vi "RGseriesSerialTest_voltage2.vi"() -> ()   [LabVIEW 2015]
uses:
  <vilib>/Platform/TimedLoop/XDataNode/timing_clust.ctl
  <vilib>/Platform/TimedLoop/XDataNode/nitl_modes.ctl
  <vilib>/Platform/TimedLoop/XDataNode/wakeup.ctl
  <vilib>/Instr/_visa.llb/VISA Configure Serial Port (Instr).vi
  <vilib>/platform/TimedLoop/XDataNode/XDataNode.xnode
  <vilib>/Platform/TimedLoop/XDataNode/XDNodeRunTimeDep.lvlib
panel:
  out "read buffer":string
  in  "Imax":dbl=1.0
  in  "stop":bool
  out "return count 8":u32
  out "return count 7":u32
  out "return count 6":u32
  out "return count 5":u32
  out "ICN MES A":dbl
  out "VCN MES V":dbl
  out "return count 4":u32
  out "return count 3":u32
  out "return count 2":u32
  out "return count":u32
  out "VCN MES":string
  in  "VISA resource name":refnum<visa-resource-name>="COM12"
  in  "timeout (10sec)":u32=10000
  out "ICN MES":string
  out "VCN_REQ_COM":string
  out "ICN_REQ_COM":string
  in  "VCN_REQ":dbl(knob) scale=0.0..5.0
  # "COM25"
  # "COM12"
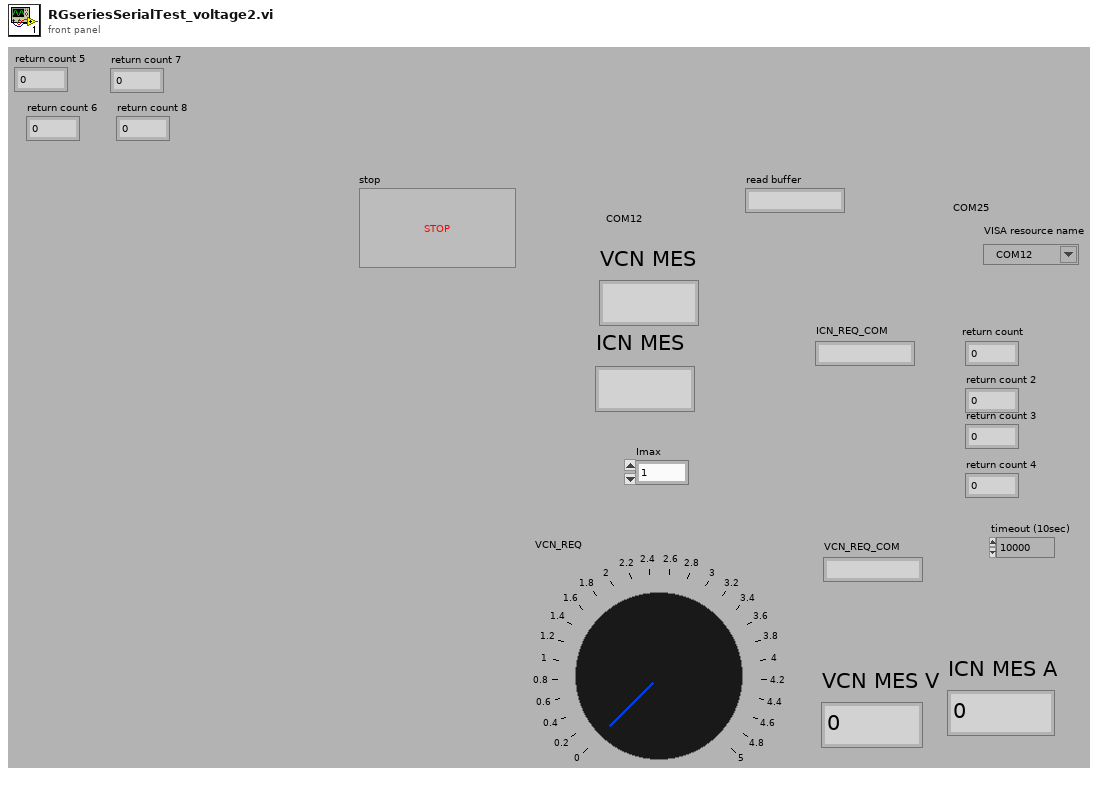
[diagram p1: front panel]
types:
  T1 = typedef "XDNodeRunTimeDep.lvlib/timing_clust.ctl" = cluster{"Expected End [f-1]":u64, "Actual End [f-1]":u64, "Finished Late? [f-1]":bool, "Expected End [i-1]":u64, "Actual End [i-1]":u64, "Finished Late? [i-1]":bool, "Expected Start [i]":u64, "Actual Start [i]":u64, "Expected Start [f]":u64, "Actual Start [f]":u64, "Source Name":string, "Structure Name":string, "Period":i64, "Deadline":i64, "Offset":i64, "Start":i64, "Priority":i32, "Timeout":i32, "Mode":T2, "Wakeup Reason":T3, "Error":errorcluster, "Source Type":string, "Secondary Source Type":string, "Global End Time":u64, "Global Start Time":u64, "Frame Duration":u64, "Iteration Duration":u64, "Assigned CPU":i32, "I/O Scan Engine Mode":u32}
  T2 = typedef "XDNodeRunTimeDep.lvlib/nitl_modes.ctl" = enum32{"No Change", "Process missed periods, maintain original phase", "Discard missed periods, maintain original phase", "Process missed periods, ignore original phase", "Discard missed periods, ignore original phase"}
  T3 = typedef "XDNodeRunTimeDep.lvlib/wakeup.ctl" = enum32{"Normal", "Aborted", "Asynchronous wakeup", "Timing source error", "Timed loop error", "Timeout"}
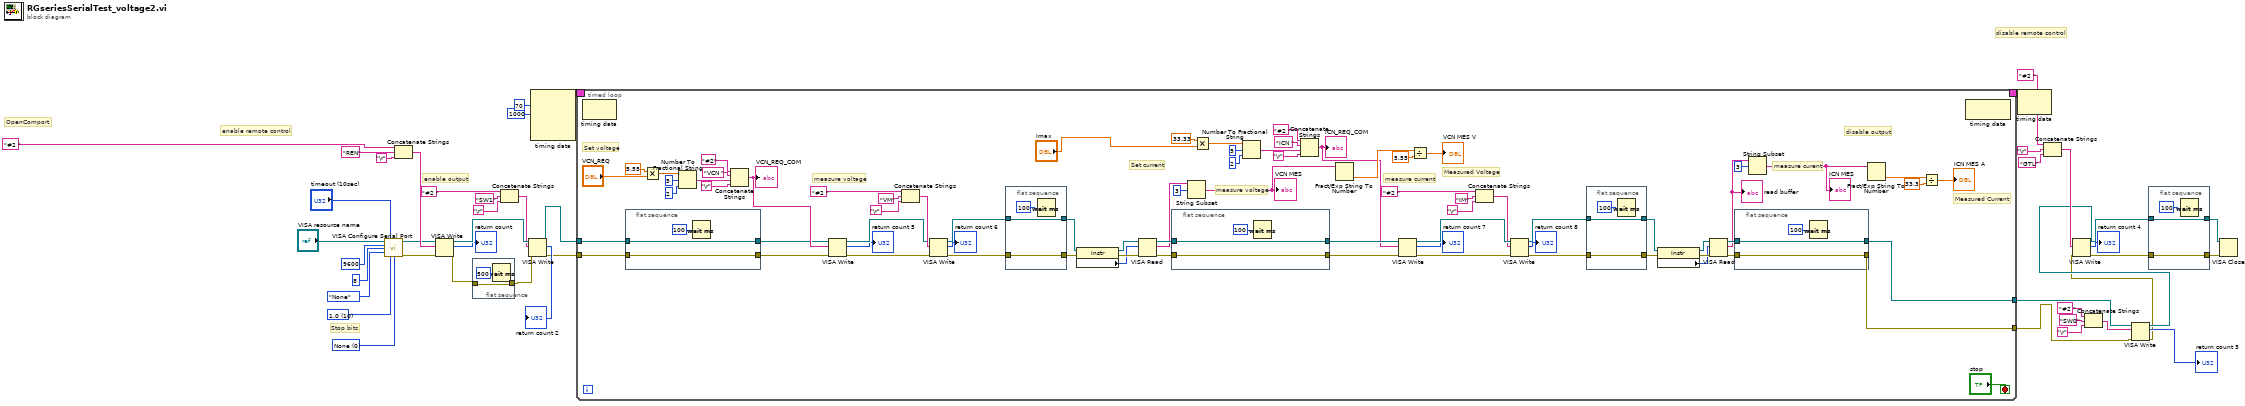
[diagram p0: block diagram]
diagram:
  w33 = u16 0 items=["None", "XON/XOFF", "RTS/CTS", "XON/XOFF & RTS/CTS", "DTR/DSR", "XON/XOFF & DTR/DSR"] ("flow control (0:none)")
  w34 = u16 10 items=["1.0"=10, "1.5"=15, "2.0"=20] ("stop bits (10: 1 bit)")
  # "OpenComport"
  # "Stop bits"
  # "enable remote control"
  # "enable output"
  # "disable remote control"
  n1 = call-poly "VISA Configure Serial Port"("VISA resource name"="VISA resource name", "timeout (10sec)"="timeout (10sec)", "baud rate (9600)"=u32 9600, "data bits (8)"=u16 8, "parity (0:none)"=enum16{"None", "Odd", "Even", "Mark", "Space"}."None", "stop bits (10: 1 bit)"=w34, "flow control (0:none)"=w33) -> ("VISA resource name out"=w28:refnum<visa-resource-name>, "error out"=w27:errorcluster)  [unwired: 7 in]
  n2 = Concatenate Strings("#2 " ("initial string"), "REN" ("string"), "\r") -> (w31:string)
  n3 = VISA Write(VISA resource name=w28, write buffer=w31, error in (no error)=w27) -> (VISA resource name out=w32:refnum<visa-resource-name>, return count=→"return count":u32, error out=w1:errorcluster)
  n4 = flat-sequence {
    tunnel: [w48] -> w2
    tunnel: w1 -> [w48]
    frame #0 {
      n5 = Wait (ms)(milliseconds to wait=u32 500) -> ()  [unwired: 1 out]
    }
  }
  n6 = Concatenate Strings("#2 " ("format string"), "SW1" ("initial string"), "\r" ("input 1")) -> (w30:string)
  n7 = VISA Write(VISA resource name=w32, write buffer=w30, error in (no error)=w2) -> (VISA resource name out=w4:refnum<visa-resource-name>, return count=→"return count 2":u32, error out=w3:errorcluster)
  n8 = node-c288(i64 1000 ("Period"), 70 ("Priority")) -> (w17:T1)  [unwired: 2 in]
  n9 = timed-loop {
    timing: w17 -> [_]
    timing-out: [_] -> w16
    tunnel: [w52] -> w6
    tunnel: [w51] -> w5
    tunnel: w4 -> [w50]
    tunnel: w3 -> [w49]
    stop <- "stop" stop-if-true
    # "measure current"
    # "measure voltage"
    # "measure voltage"
    # "measure curent"
    # "Measured Voltage"
    # "Measured Current"
    # "Set current"
    # "Set voltage"
    # "disable output"
    n10 = node-c288() -> ()  [unwired: 1 in, 1 out]
    n11 = flat-sequence {
      tunnel: w50 -> [w136]
      tunnel: w49 -> [w137]
      tunnel: [w137] -> w55
      tunnel: [w136] -> w56
      frame #0 {
        n12 = Wait (ms)(milliseconds to wait=u32 100) -> ()  [unwired: 1 out]
      }
    }
    n13 = Multiply(x=5.55, y="VCN_REQ") -> (x*y=w120:dbl)
    n14 = Number To Fractional String(number=w120, width (-)=i16 5, precision (6)=i16 2) -> (F-format string=w122:string)  [unwired: 1 in]
    n15 = Concatenate Strings("#2" ("format string"), "VCN " ("initial string"), w122, "\r") -> (w60:string)
    "VCN_REQ_COM" <- w60
    n16 = VISA Write(VISA resource name=w56, write buffer=w60, error in (no error)=w55) -> (VISA resource name out=w94:refnum<visa-resource-name>, return count=→"return count 5":u32, error out=w93:errorcluster)
    n17 = Concatenate Strings("#2 " ("format string"), "VM" ("initial string"), "\r" ("input 1")) -> (w95:string)
    n18 = VISA Write(VISA resource name=w94, write buffer=w95, error in (no error)=w93) -> (VISA resource name out=w76:refnum<visa-resource-name>, return count=→"return count 6":u32, error out=w74:errorcluster)
    n19 = flat-sequence {
      tunnel: w76 -> [w135]
      tunnel: [w135] -> w75
      tunnel: w74 -> [w134]
      tunnel: [w134] -> w73
      frame #0 {
        n20 = Wait (ms)(milliseconds to wait=u32 100) -> ()  [unwired: 1 out]
      }
    }
    n21 = property class="Instr"(reference=w75, error in=w73) -> (reference out=w82:refnum<visa-resource-name>, error out=w81:errorcluster, "Serial Settings:Number of Bytes at Serial Port"=w80:u32)
    n22 = VISA Read(VISA resource name=w82, byte count=w80, error in (no error)=w81) -> (VISA resource name out=w68:refnum<visa-resource-name>, read buffer=w61:string, error out=w67:errorcluster)  [unwired: 1 out]
    n23 = flat-sequence {
      tunnel: w68 -> [w128]
      tunnel: w67 -> [w127]
      tunnel: [w128] -> w65
      tunnel: [w127] -> w66
      frame #0 {
        n24 = Wait (ms)(milliseconds to wait=u32 100) -> ()  [unwired: 1 out]
      }
    }
    n25 = String Subset(string=w61, offset (0)=3) -> (substring=w58:string)  [unwired: 1 in]
    "VCN MES" <- w58
    n26 = Multiply(x=33.33, y="Imax") -> (x*y=w110:dbl)
    n27 = Number To Fractional String(number=w110, width (-)=i16 5, precision (6)=i16 2) -> (F-format string=w113:string)  [unwired: 1 in]
    n28 = Concatenate Strings("#2 " ("initial string"), "ICN " ("initial string"), w113, "\r") -> (w59:string)
    "ICN_REQ_COM" <- w59
    n29 = Fract/Exp String To Number(string=w58) -> (number=w104:dbl)  [unwired: 3 in, 1 out]
    n30 = VISA Write(VISA resource name=w65, write buffer=w59, error in (no error)=w66) -> (VISA resource name out=w90:refnum<visa-resource-name>, return count=→"return count 7":u32, error out=w91:errorcluster)
    n31 = Divide(x=w104, y=5.55 ("x")) -> (x/y=→"VCN MES V":dbl)
    n32 = Concatenate Strings("#2 " ("format string"), "IM" ("initial string"), "\r" ("input 1")) -> (w88:string)
    n33 = VISA Write(VISA resource name=w90, write buffer=w88, error in (no error)=w91) -> (VISA resource name out=w72:refnum<visa-resource-name>, return count=→"return count 8":u32, error out=w71:errorcluster)
    n34 = flat-sequence {
      tunnel: w72 -> [w131]
      tunnel: w71 -> [w130]
      tunnel: [w131] -> w70
      tunnel: [w130] -> w69
      frame #0 {
        n35 = Wait (ms)(milliseconds to wait=u32 100) -> ()  [unwired: 1 out]
      }
    }
    n36 = property class="Instr"(reference=w70, error in=w69) -> (reference out=w79:refnum<visa-resource-name>, error out=w78:errorcluster, "Serial Settings:Number of Bytes at Serial Port"=w77:u32)
    n37 = VISA Read(VISA resource name=w79, byte count=w77, error in (no error)=w78) -> (VISA resource name out=w64:refnum<visa-resource-name>, read buffer=w62:string, error out=w63:errorcluster)  [unwired: 1 out]
    "read buffer" <- w62
    n38 = flat-sequence {
      tunnel: w64 -> [w125]
      tunnel: w63 -> [w124]
      tunnel: [w125] -> w52
      tunnel: [w124] -> w51
      frame #0 {
        n39 = Wait (ms)(milliseconds to wait=u32 100) -> ()  [unwired: 1 out]
      }
    }
    n40 = String Subset(string=w62, offset (0)=3) -> (substring=w57:string)  [unwired: 1 in]
    "ICN MES" <- w57
    n41 = Fract/Exp String To Number(string=w57) -> (number=w101:dbl)  [unwired: 3 in, 1 out]
    n42 = Divide(x=w101, y=33.3 ("x")) -> (x/y=→"ICN MES A":dbl)
    n43 = node-c288() -> ()  [unwired: 1 in, 1 out]
  }
  n44 = node-c288(w16) -> ()  [unwired: 1 out]
  n45 = Concatenate Strings("#2 " ("initial string"), "\r", "GTL" ("input 1")) -> (w29:string)
  n46 = Concatenate Strings("#2 " ("format string"), "SW0" ("initial string"), "\r" ("input 1")) -> (w13:string)
  n47 = VISA Write(VISA resource name=w6, write buffer=w13, error in (no error)=w5) -> (VISA resource name out=w8:refnum<visa-resource-name>, return count=→"return count 3":u32, error out=w7:errorcluster)
  n48 = VISA Write(VISA resource name=w8, write buffer=w29, error in (no error)=w7) -> (VISA resource name out=w20:refnum<visa-resource-name>, return count=→"return count 4":u32, error out=w21:errorcluster)
  n49 = flat-sequence {
    tunnel: w20 -> [w142]
    tunnel: w21 -> [w141]
    tunnel: [w142] -> w19
    tunnel: [w141] -> w18
    frame #0 {
      n50 = Wait (ms)(milliseconds to wait=u32 100) -> ()  [unwired: 1 out]
    }
  }
  n51 = VISA Close(VISA resource name=w19, error in (no error)=w18) -> ()  [unwired: 1 out]
